vi "Ramp to Set.vi"(8 "error in (no error)":errorcluster, 11 "Instrument.1820 in":refnum<class "Instrument.Oxford1820.lvclass">) -> (0 "error out":errorcluster, 2 "Response":string, 3 "Instrument.1820 in":refnum<class "Instrument.Oxford1820.lvclass">)   [LabVIEW 2019, in "Instrument.Oxford1820.lvclass"]
uses:
  Instrument.Oxford1820.lvclass
  C:/Program Files (x86)/National Instruments/LabVIEW 2019/user.lib/LevyLab/Instrument Framework/Instrument/Instrument.lvclass
  <instrlib>/Mercury iXX/Public/Libraries/Magnet/Controls/PSU Actions.ctl
  Typedefs/Instrument.Oxford1820.Commands-enum.ctl
  1cef2048-2a77-4234-8fe1-be5101f2e318.vi
  1cef2048-2a77-4234-8fe1-be5101f2e318.vi/1e386510-6aca-44ce-897a-d265b21b0e25.vi
  1cef2048-2a77-4234-8fe1-be5101f2e318.vi/1e386510-6aca-44ce-897a-d265b21b0e25.vi/92e266c3-c1c2-49a7-90da-b3875889a329.vi
  1cef2048-2a77-4234-8fe1-be5101f2e318.vi/1e386510-6aca-44ce-897a-d265b21b0e25.vi/c5e54412-6348-496c-86c0-fde1c829c2b3.vi
  <userlib>/LevyLab/Instrument Framework/Instrument/API/RemoteClient.vi
  <vilib>/Utility/Data Type/Get Type Information.vi
  <vilib>/JDP Science/JSONtext/JSON text to Variant.vi
  <vilib>/JDP Science/JSONtext/LVClass Serializer/JSONtext LVClass Serializer.lvclass
  <instrlib>/Mercury iXX/Public/Libraries/Magnet.lvlib
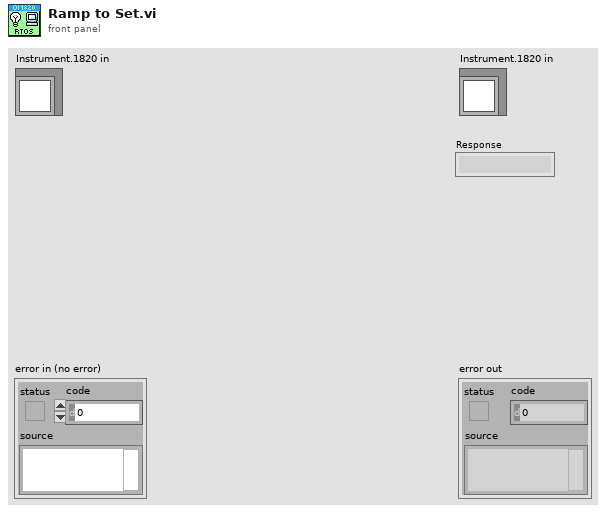
[diagram p1: front panel]
types:
  T1 = typedef "Instrument.Oxford1820.lvclass/Instrument.Oxford1820.Commands-enum.ctl" = enum16{"setAction", "setTarget", "setSwitchHeat", "setLambda", "setFillMode", "setNeedleValve", "setMagnetField", "getStatus", "getTarget", "getSwitchHeat", "getPSUField", "setSequenceStatus", "getMagnetField"}
  T2 = typedef "Mercury iXX.lvlib/Magnet.lvlib/PSU Actions.ctl" = string
  T3 = cluster{"Holding":bool, "Ramp to Setpoint":bool, "Ramp to Zero":bool, "Clamp":bool}
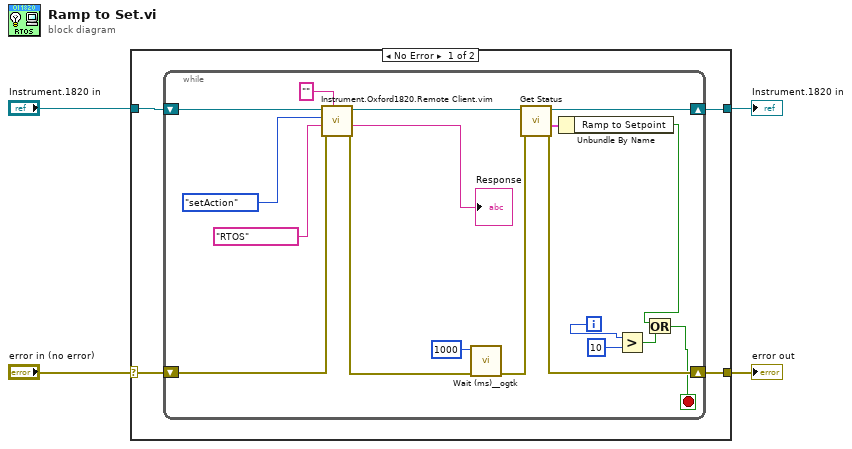
[diagram p0: block diagram]
diagram:
  n1 = case shown="No Error" "error in (no error)" {
    selector: "error in (no error)" -> [w7 w28]
    tunnel: [w6 w28] -> w3
    tunnel: [w5 w27] -> w1
    tunnel: "Instrument.1820 in" -> [w8 w27]
    frame No Error {
      n2 = while {
        shift-right: [w19] -> w5
        shift-left: w8 -> [w18]
        shift-right: [w20] -> w6
        shift-left: w7 -> [w24]
        i -> [w13]
        stop <- w14 stop-if-true
        n3 = call "Instrument.Oxford1820.Remote Client.vim"("Data Out type"="", "error in (no error)"=w24, "Data"=T2 "RTOS" ("PSU Act Stat"), "Commands"=Instrument.Oxford1820.Commands-enum."setAction", "Instrument.1820 in"=w18) -> ("error out"=w9:errorcluster, "Data out"=→"Response":string, "Instrument.1820 out"=w11:refnum<class "Instrument.Oxford1820.lvclass">)  [unwired: 4 in]
        n4 = call <userlib>:"Wait (ms)__ogtk.vi"("error in (no error)"=w9, "milliseconds to wait"=u32 1000) -> ("error out"=w21:errorcluster)  [unwired: 8 in, 1 out]
        n5 = call "Get Status.vi"("error in (no error)"=w21, "Instrument.1820 in"=w11) -> ("error out"=w20:errorcluster, "Status"=w22:T3, "Instrument.1820 in"=w19:refnum<class "Instrument.Oxford1820.lvclass">)  [unwired: 6 in, 1 out]
        n6 = Unbundle By Name(w22) -> ("Ramp to Setpoint"=w15:bool)
        n7 = Greater?(x=w13, y=10) -> (0:w16:bool)
        n8 = Or(x=w15, y=w16) -> (x .or. y?=w14:bool)
      }
    }
    frame Error {
    }
  }
  "error out" <- w3
  "Instrument.1820 in" <- w1
